vi "Get SubPicture Coordinate.vi"(11 "Image in":u32[](array[numeric])) -> (3 "quotient":i32)   [LabVIEW 2020, in "lv_icon.lvlib"]
doc: "Get sub-coordinates to the pixel."
uses:
  <vilib>/LabVIEW Icon API/lv_icon/lv_icon.lvlib
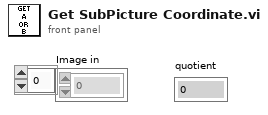
[diagram p1: front panel]
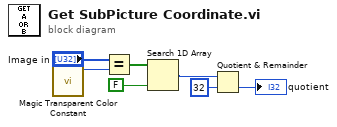
[diagram p0: block diagram]
diagram:
  n1 = call <vilib>:"Magic Transparent Color Constant.vi"() -> ("Magic transparent color constant"=w2:u32)  [unwired: 11 out]
  n2 = Equal?(x="Image in", y=w2) -> (x = y?=w3:bool[])
  n3 = Search 1D Array(1D array=w3, element=FALSE) -> (index of element=w6:i32)  [unwired: 1 out]
  n4 = Quotient & Remainder(x=w6, y=32) -> (floor(x/y)=→"quotient":i32)  [unwired: 1 out]
